vi "Open Spreadsheet File (Consequtive Delimeters).vi"(11 "File":path caption="Spreadsheet File") -> (3 "Array":string[][](array[string])=[["T", "F", "6", "3", "3", "0", "6", "6", "6", "6", "6", "6", "1", "0", "0", "0.0000.00000", ""], ["0", "1", "1", "0", "0", "0", "0.00000", "0.00000", "0.00000", "0.00000", "0.00000", "", "", "", "", "", ""], ["-99.000", "-99.000", "-99.000", "", "", "", "", "", "", "", "", "", "", "", "", "", ""], ["-99.00000", "-99.00000", "-99.00000", "1.416445", "0.000736", "!", "H2O", "&", "O3", "COLUMNS", "[GM/CM2]", "", "", "", "", "", ""], ["361976", "U", "S", "STANDARD", "", "", "", "", "", "", "", "", "", "", "", "", ""], ["2.00000", "100.00000", "0.00000", "98.00000", "0.000006371.00000", "0", "0.00000", "", "", "", "", "", "", "", "", "", ""], ["-99", "-99", "1", "0", "", "", "", "", "", "", "", "", "", "", "", "", ""], ["-99.00000", "-99.00000", "-99.00000", "-99.00000", "-99.00000", "-99.00000", "0.00000", "-99.00000", "", "", "", "", "", "", "", "", ""], ["833.0", "1250.0", "10.0", "1.0RM,", "", "", "", "", "", "", "", "", "", "", "", "", ""], ["0", "0", "0.000", "0", "0.000", "0", "1.000", "", "", "", "", "", "", "", "", "", ""], ["FREQ", "TRANS", "SOL", "TR", "SOLAR", "", "", "", "", "", "", "", "", "", "", "", ""], ["833.00", "0.9705", "1.73E-07", "1.78E-07", "2.996E-02", "", "", "", "", "", "", "", "", "", "", "", ""], ["843.00", "0.9657", "1.76E-07", "1.82E-07", "3.489E-02", "", "", "", "", "", "", "", "", "", "", "", ""], ["853.00", "0.7844", "1.46E-07", "1.86E-07", "2.428E-01", "", "", "", "", "", "", "", "", "", "", "", ""], ["863.00", "0.9737", "1.86E-07", "1.91E-07", "2.668E-02", "", "", "", "", "", "", "", "", "", "", "", ""], ["873.00", "0.9720", "1.89E-07", "1.95E-07", "2.840E-02", "", "", "", "", "", "", "", "", "", "", "", ""], ["883.00", "0.9576", "1.91E-07", "1.99E-07", "4.334E-02", "", "", "", "", "", "", "", "", "", "", "", ""], ["893.00", "0.9731", "1.98E-07", "2.04E-07", "2.725E-02", "", "", "", "", "", "", "", "", "", "", "", ""], ["903.00", "0.9756", "2.03E-07", "2.08E-07", "2.470E-02", "", "", "", "", "", "", "", "", "", "", "", ""], ["913.00", "0.9724", "2.07E-07", "2.13E-07", "2.797E-02", "", "", "", "", "", "", "", "", "", "", "", ""], ["923.00", "0.9594", "2.08E-07", "2.17E-07", "4.143E-02", "", "", "", "", "", "", "", "", "", "", "", ""], ["933.00", "0.9637", "2.14E-07", "2.22E-07", "3.702E-02", "", "", "", "", "", "", "", "", "", "", "", ""], ["943.00", "0.9792", "2.22E-07", "2.27E-07", "2.097E-02", "", "", "", "", "", "", "", "", "", "", "", ""], ["953.00", "0.9231", "2.13E-07", "2.31E-07", "8.000E-02", "", "", "", "", "", "", "", "", "", "", "", ""], ["963.00", "0.9720", "2.29E-07", "2.36E-07", "2.840E-02", "", "", "", "", "", "", "", "", "", "", "", ""], ["973.00", "0.9253", "2.23E-07", "2.41E-07", "7.760E-02", "", "", "", "", "", "", "", "", "", "", "", ""], ["983.00", "0.9558", "2.35E-07", "2.46E-07", "4.516E-02", "", "", "", "", "", "", "", "", "", "", "", ""], ["993.00", "0.9173", "2.30E-07", "2.50E-07", "8.628E-02", "", "", "", "", "", "", "", "", "", "", "", ""], ["1003.00", "0.7966", "2.03E-07", "2.55E-07", "2.274E-01", "", "", "", "", "", "", "", "", "", "", "", ""], ["1013.00", "0.6272", "1.63E-07", "2.60E-07", "4.664E-01", "", "", "", "", "", "", "", "", "", "", "", ""], ["1023.00", "0.4086", "1.08E-07", "2.65E-07", "8.950E-01", "", "", "", "", "", "", "", "", "", "", "", ""], ["1033.00", "0.4100", "1.11E-07", "2.70E-07", "8.915E-01", "", "", "", "", "", "", "", "", "", "", "", ""], ["1043.00", "0.8178", "2.25E-07", "2.75E-07", "2.012E-01", "", "", "", "", "", "", "", "", "", "", "", ""], ["1053.00", "0.3112", "8.73E-08", "2.80E-07", "1.167E+00", "", "", "", "", "", "", "", "", "", "", "", ""], ["1063.00", "0.5303", "1.51E-07", "2.86E-07", "6.343E-01", "", "", "", "", "", "", "", "", "", "", "", ""], ["1073.00", "0.8887", "2.59E-07", "2.91E-07", "1.180E-01", "", "", "", "", "", "", "", "", "", "", "", ""], ["1083.00", "0.9308", "2.76E-07", "2.96E-07", "7.174E-02", "", "", "", "", "", "", "", "", "", "", "", ""], ["1093.00", "0.9496", "2.86E-07", "3.01E-07", "5.167E-02", "", "", "", "", "", "", "", "", "", "", "", ""], ["1103.00", "0.9598", "2.95E-07", "3.07E-07", "4.103E-02", "", "", "", "", "", "", "", "", "", "", "", ""], ["1113.00", "0.9546", "2.98E-07", "3.12E-07", "4.649E-02", "", "", "", "", "", "", "", "", "", "", "", ""], ["1123.00", "0.9568", "3.04E-07", "3.18E-07", "4.414E-02", "", "", "", "", "", "", "", "", "", "", "", ""], ["1133.00", "0.9487", "3.07E-07", "3.23E-07", "5.265E-02", "", "", "", "", "", "", "", "", "", "", "", ""], ["1143.00", "0.9537", "3.13E-07", "3.29E-07", "4.739E-02", "", "", "", "", "", "", "", "", "", "", "", ""], ["1153.00", "0.8858", "2.96E-07", "3.34E-07", "1.212E-01", "", "", "", "", "", "", "", "", "", "", "", ""], ["1163.00", "0.9458", "3.22E-07", "3.40E-07", "5.573E-02", "", "", "", "", "", "", "", "", "", "", "", ""], ["1173.00", "0.8941", "3.09E-07", "3.46E-07", "1.120E-01", "", "", "", "", "", "", "", "", "", "", "", ""], ["1183.00", "0.9455", "3.32E-07", "3.51E-07", "5.600E-02", "", "", "", "", "", "", "", "", "", "", "", ""], ["1193.00", "0.9479", "3.38E-07", "3.57E-07", "5.347E-02", "", "", "", "", "", "", "", "", "", "", "", ""], ["1203.00", "0.9657", "3.50E-07", "3.63E-07", "3.490E-02", "", "", "", "", "", "", "", "", "", "", "", ""], ["1213.00", "0.7355", "2.71E-07", "3.69E-07", "3.072E-01", "", "", "", "", "", "", "", "", "", "", "", ""], ["1223.00", "0.8238", "3.09E-07", "3.75E-07", "1.938E-01", "", "", "", "", "", "", "", "", "", "", "", ""], ["1233.00", "0.8867", "3.38E-07", "3.81E-07", "1.203E-01", "", "", "", "", "", "", "", "", "", "", "", ""], ["1243.00", "0.4994", "1.93E-07", "3.87E-07", "6.943E-01", "", "", "", "", "", "", "", "", "", "", "", ""], ["-9999.", "", "", "", "", "", "", "", "", "", "", "", "", "", "", "", ""]])   [LabVIEW 2010]
uses:
  <vilib>/Utility/file.llb/Read From Spreadsheet File (string).vi
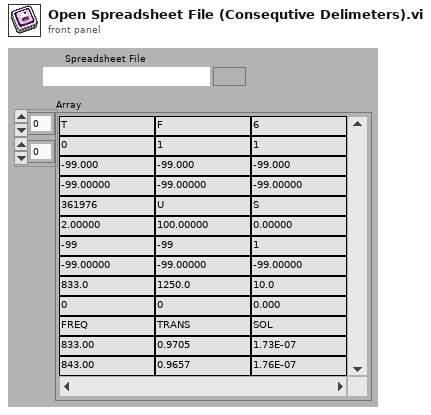
[diagram p1: front panel]
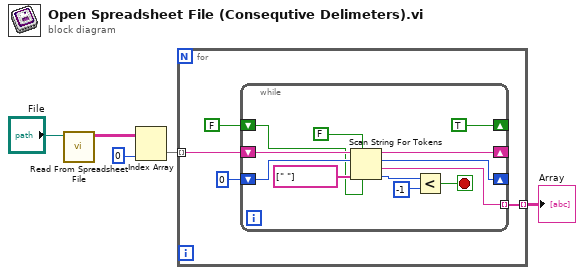
[diagram p0: block diagram]
diagram:
  n1 = call-poly <vilib>:"Read From Spreadsheet File.vi"("file path (dialog if empty)"="File") -> ("all rows"=w3:string[][])  [unwired: 6 in, 4 out]
  n2 = Index Array(array=w3, index (col)=0 ("disabled index (col)")) -> (element=w2:string[])  [unwired: 1 in]
  n3 = for {
    tunnel: w2 -> [w9] mode=indexing
    tunnel: [w8] -> w4 mode=indexing
    n4 = while {
      shift-right: [w19] -> _
      shift-left: w9 -> [w20]
      tunnel: [w17] -> w8 mode=indexing
      shift-right: [w16] -> _
      shift-left: 0 ("offset past token") -> [w15]
      shift-right: [TRUE ("allow empty tokens? (F)")] -> _
      shift-left: FALSE ("allow empty tokens? (F)") -> [w11]
      stop <- w12 stop-if-true
      n5 = Scan String For Tokens(4:w11, 5:FALSE ("allow empty tokens? (F)"), 6:string[] [" "] ("delimiters (\\s,\\t,\\r,\\n)"), 8:w15, 9:w20) -> (0:w14:i32, 1:w17:string, 2:w16:i32, 3:w19:string)  [unwired: 1 in]
      n6 = Less?(x=w14, y=-1) -> (x < y?=w12:bool)
    }
  }
  "Array" <- w4
